vi "Bamocar Serial.vi"(8 "Error In":errorcluster, 9 "Register":T1 items=["Motor temp warning threshold"=162, "Motor temp fault threshold"=163, "Drive Enable"=81], 10 "Value to write":u16, 11 "Command":enum16{"Write/Read", "Write", "Read"}(ring)=enum."Read") -> (0 "Error Out":errorcluster, 3 "Decimal":u32)   [LabVIEW 2018]
uses:
  TypeDefs/bamocarRegisters.ctl
  <vilib>/Instr/_visa.llb/VISA Configure Serial Port (Instr).vi
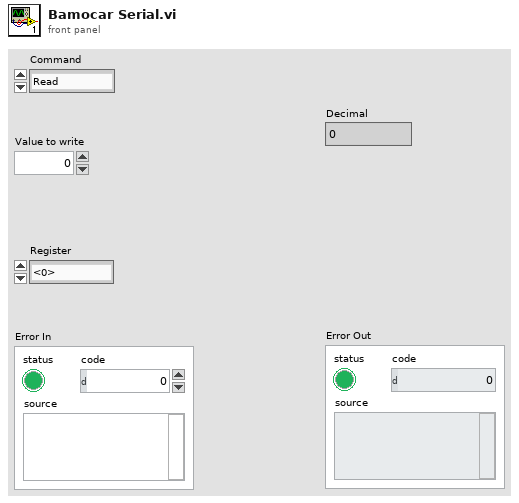
[diagram p1: front panel]
types:
  T1 = typedef "bamocarRegisters.ctl" = u16
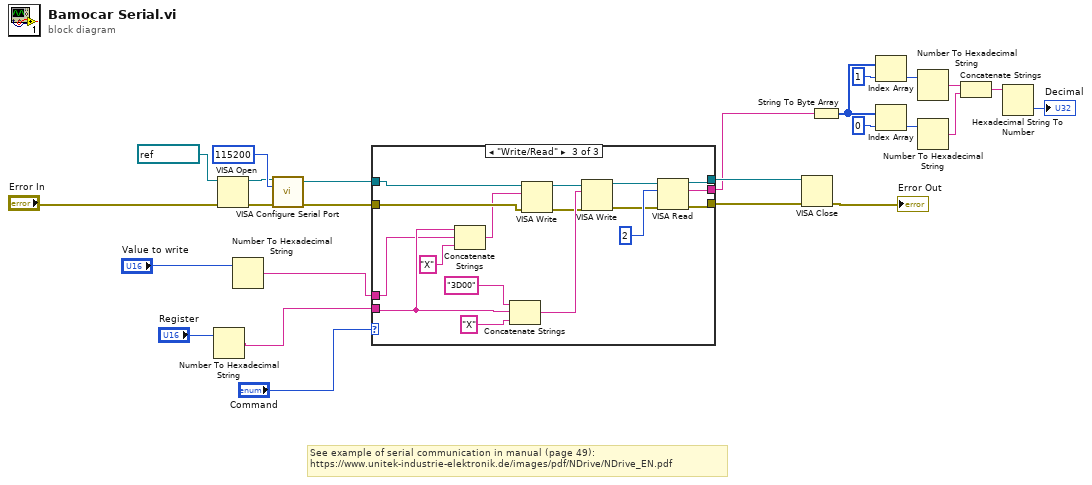
[diagram p0: block diagram]
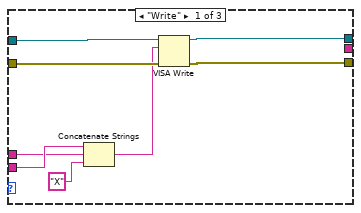
[diagram p2: hidden frame]
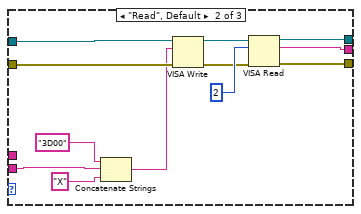
[diagram p3: hidden frame]
diagram:
  # "See example of serial communication in manual (page 49):\nhttps://www.unitek-industrie-elektronik.de/images/pdf/NDrive/NDrive_EN.pdf"
  n1 = Number To Hexadecimal String(2:"Register") -> (0:w5:string)  [unwired: 1 in]
  n2 = VISA Open(error in (no error)="Error In", VISA resource name=refnum<visa-resource-name> "COM3") -> (VISA resource name=w23:refnum<visa-resource-name>, error out=w24:errorcluster)  [unwired: 3 in]
  n3 = Number To Hexadecimal String(2:"Value to write") -> (0:w2:string)  [unwired: 1 in]
  n4 = call-poly "VISA Configure Serial Port"("VISA resource name"=w23, "baud rate (9600)"=u32 115200, "error in (no error)"=w24) -> ("VISA resource name out"=w10:refnum<visa-resource-name>, "error out"=w11:errorcluster)  [unwired: 11 in]
  n5 = case shown="\"Write/Read\"" "Command" {
    tunnel: w5 -> [w33 w44 w47]
    tunnel: w2 -> [w32 _ w46]
    tunnel: w11 -> [w29 w42 w51]
    tunnel: w10 -> [w30 w40 w50]
    tunnel: [w27 w36 w56] -> w9
    tunnel: [w26 w35 w55] -> w8
    tunnel: [_ w34 w54] -> w7
    frame "Write" {
      n6 = Concatenate Strings(w33, w32, "X" ("string")) -> (w28:string)
      n7 = VISA Write(VISA resource name=w30, write buffer=w28, error in (no error)=w29) -> (VISA resource name out=w26:refnum<visa-resource-name>, error out=w27:errorcluster)  [unwired: 1 out]
    }
    frame "Read", Default {
      n8 = Concatenate Strings("3D00" ("string"), w44, "X" ("string")) -> (w41:string)
      n9 = VISA Write(VISA resource name=w40, write buffer=w41, error in (no error)=w42) -> (VISA resource name out=w37:refnum<visa-resource-name>, error out=w38:errorcluster)  [unwired: 1 out]
      n10 = VISA Read(VISA resource name=w37, byte count=u32 2, error in (no error)=w38) -> (VISA resource name out=w35:refnum<visa-resource-name>, read buffer=w34:string, error out=w36:errorcluster)  [unwired: 1 out]
    }
    frame "Write/Read" {
      n11 = Concatenate Strings(w47, w46, "X" ("string")) -> (w48:string)
      n12 = Concatenate Strings("3D00" ("string"), w47, "X" ("string")) -> (w60:string)
      n13 = VISA Write(VISA resource name=w50, write buffer=w48, error in (no error)=w51) -> (VISA resource name out=w52:refnum<visa-resource-name>, error out=w53:errorcluster)  [unwired: 1 out]
      n14 = VISA Write(VISA resource name=w52, write buffer=w60, error in (no error)=w53) -> (VISA resource name out=w57:refnum<visa-resource-name>, error out=w58:errorcluster)  [unwired: 1 out]
      n15 = VISA Read(VISA resource name=w57, byte count=u32 2, error in (no error)=w58) -> (VISA resource name out=w55:refnum<visa-resource-name>, read buffer=w54:string, error out=w56:errorcluster)  [unwired: 1 out]
    }
  }
  n16 = VISA Close(VISA resource name=w8, error in (no error)=w9) -> (error out=→"Error Out":errorcluster)
  n17 = String To Byte Array(string=w7) -> (unsigned byte array=w17:u8[])
  n18 = Index Array(array=w17, index=1) -> (element=w19:u8)
  n19 = Index Array(array=w17, index=0) -> (element=w16:u8)
  n20 = Number To Hexadecimal String(2:w19) -> (0:w15:string)  [unwired: 1 in]
  n21 = Number To Hexadecimal String(2:w16) -> (0:w12:string)  [unwired: 1 in]
  n22 = Concatenate Strings(w15, w12) -> (w14:string)
  n23 = Hexadecimal String To Number(string=w14) -> (number=→"Decimal":u32)  [unwired: 2 in, 1 out]
